vi "enqueueAll.vi"(8 "Waypoint Queue":refnum<queue>, 10 "timeout in ms (-1)":i32, 11 "Waypoint Array":refnum<class "Waypoint.lvclass">[](array[class])) -> (3 "Waypoint Queue Out":refnum<queue>)   [LabVIEW 2013]
doc: "Takes an array of elements and add all to the queue, starting with E0 and ending with En"
uses:
  Logic/Classes/Waypoint/Waypoint.lvclass
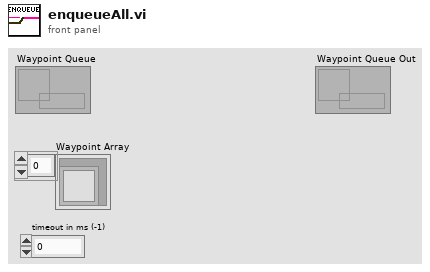
[diagram p1: front panel]
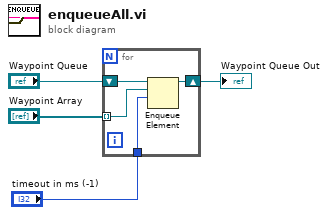
[diagram p0: block diagram]
diagram:
  n1 = for {
    shift-right: [w8] -> w4
    shift-left: "Waypoint Queue" -> [w7]
    tunnel: "Waypoint Array" -> [w6] mode=indexing
    tunnel: "timeout in ms (-1)" -> [w5]
    n2 = Enqueue Element(queue=w7, element=w6, timeout in ms (-1)=w5) -> (queue out=w8:refnum<queue>)  [unwired: 1 in, 2 out]
  }
  "Waypoint Queue Out" <- w4
